vi "LoadPressureAndTangents.vi"(4 "error in (no error)":errorcluster, 5 "Red Graph":refnum<vi>, 6 "ResetFrontImage":bool, 7 "Blue Graph":refnum<vi>) -> (0 "error out":errorcluster, 3 "output cluster":cluster{dbl, dbl, dbl, dbl})   [LabVIEW 2013, in "main.lvlib"]
uses:
  main.lvlib
  Controls/Enum Process Data.ctl
  Controls/Combobox Filename.ctl
  Controls/Enum Variables.ctl
  <userlib>/_OpenG.lib/file/file.llb/File Exists - Scalar__ogtk.vi
  <vilib>/Utility/file.llb/Read From Spreadsheet File (DBL).vi
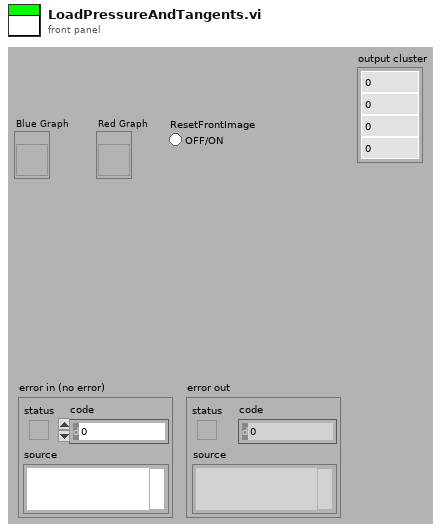
[diagram p1: front panel]
types:
  T1 = typedef "main.lvlib/Enum Variables.ctl" = enum16{"SetAcqFilter", "GetAcqFilter", "Set Filter", "Get Filter", "Set Height", "Get Height", "Set Recorded Height", "Get Recorded Height", "Set Blue Pressure", "Get Blue Pressure", "Set Red Pressure", "Get Red Pressure", "Init", "Reset Pressure", "Set Red Cursors", "Get Red Cursors", "Set Blue Cursors", "Get Blue Cursors", "Set Language", "Get Language", "Set Active Graphs", "Get ActiveGraphs", "Set Method", "Get Method", "Set Encryption", "Get Encryption", "Set ExcelVersion", "Get ExcelVersion", "Set DICOM Avail", "Get DICOM Avail", "Set DICOM Encode", "Get DICOM Encode", "Set JournalExport", "Get JournalExport", "Set Sequence", "Get Sequence", "Set DAQ Connected", "Get DAQ Connected", "Set Current Graph", "Get Current Graph", "Set General Settings", "Get Hyphenation", "Set Arm Calc Method", "Get Arm Calc Method", "Set Dicom Tags", "Get Dicom Tags", "Set BT Serial", "Get BT Serial", "Set BT Accepted Serials", "Get BT Accepted Serials", "Get BT License", "Set BT License"}
  T2 = typedef "main.lvlib/Combobox Filename.ctl" = string
  T3 = typedef "main.lvlib/Enum Process Data.ctl" = enum16{"Init", "Set Cursor Mode", "Set Data Path", "Get All"}
  T4 = cluster{dbl, dbl, "Armpressure":dbl, "Armpressure":dbl}
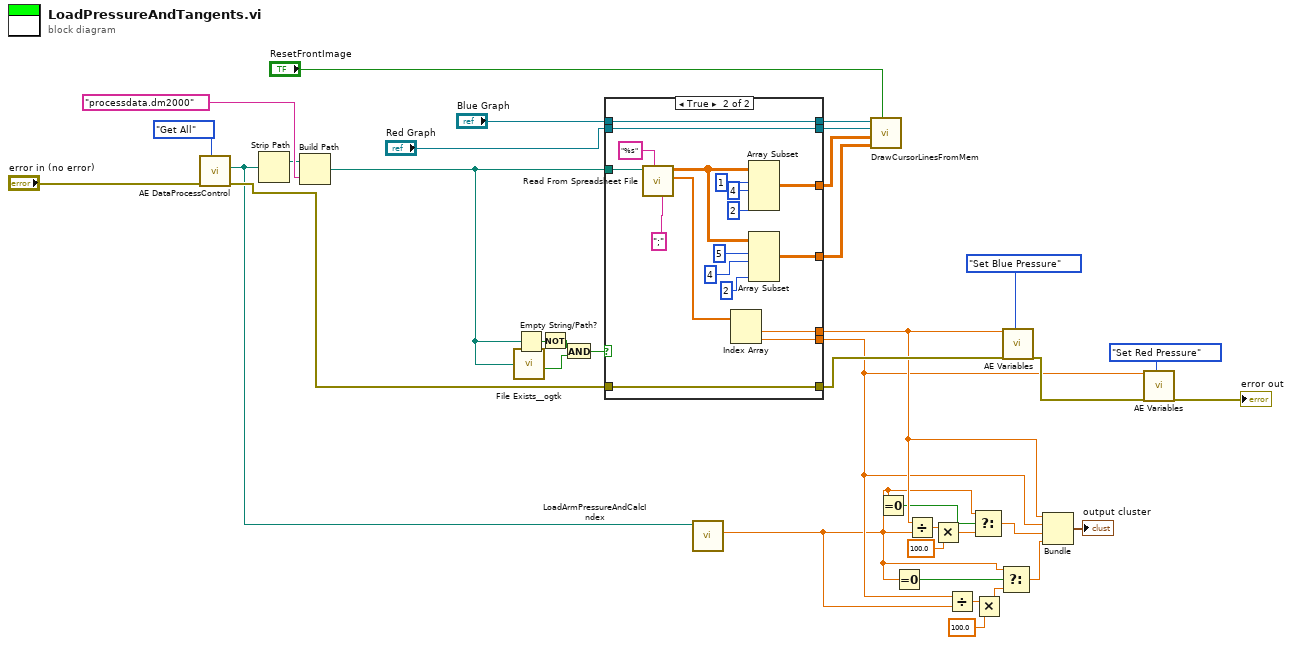
[diagram p0: block diagram]
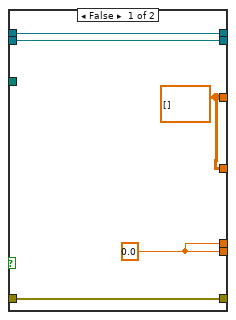
[diagram p2: hidden frame]
diagram:
  n1 = call "AE DataProcessControl.vi"("Action"=Enum_Process_Data."Get All", "error in (no error)"="error in (no error)") -> ("error out"=w25:errorcluster, "Data Path Out"=w21:path)  [unwired: 7 in, 1 out]
  n2 = Strip Path(path=w21) -> (stripped path=w28:path)  [unwired: 1 out]
  n3 = Build Path(base path=w28, name or relative path=T2 "processdata.dm2000" ("FileName")) -> (appended path=w1:path)
  n4 = call-poly <userlib>:"File Exists__ogtk.vi"("file path"=w1) -> ("exists"=w3:bool)  [unwired: 6 in, 1 out]
  n5 = Empty String/Path?(string/path=w1) -> (empty?=w5:bool)
  n6 = Not(x=w5) -> (.not. x?=w4:bool)
  n7 = And(x=w4, y=w3) -> (x .and. y?=w2:bool)
  n8 = case shown="True" w2 {
    tunnel: w1 -> [_ w57]
    tunnel: [w42 w56] -> w15
    tunnel: [w42 w55] -> w18
    tunnel: [w41 w51] -> w32
    tunnel: [w41 w49] -> w33
    tunnel: [w40 w45] -> w35
    tunnel: "Blue Graph" -> [w40 w45]
    tunnel: "Red Graph" -> [w39 w44]
    tunnel: [w39 w44] -> w36
    tunnel: w25 -> [w38 w43]
    tunnel: [w38 w43] -> w24
    frame False {
      w41 = dbl[][] []
      w42 = 0.0
    }
    frame True {
      n9 = call-poly <vilib>:"Read From Spreadsheet File.vi"("delimiter (\\t)"=";" ("delimiter (\\t)"), "format (%.3f)"="%s", "file path (dialog if empty)"=w57) -> ("first row"=w58:dbl[], "all rows"=w50:dbl[][])  [unwired: 4 in, 3 out]
      n10 = Index Array(array=w58) -> (element #1=w55:dbl, element #2=w56:dbl)  [unwired: 2 in]
      n11 = Array Subset(array=w50, index (row)=1 ("index"), length (row)=4 ("length"), length (col)=2 ("length")) -> (w51:dbl[][])  [unwired: 1 in]
      n12 = Array Subset(array=w50, index (row)=5 ("index"), length (row)=4 ("length"), length (col)=2 ("length")) -> (w49:dbl[][])  [unwired: 1 in]
    }
  }
  n13 = call "LoadArmPressureAndCalcIndex.vi"("Path"=w21) -> ("Armpressure"=w8:dbl)  [unwired: 8 in, 2 out]
  n14 = call "DrawCursorLinesFromMem.vi"("CursorMode"="ResetFrontImage", "RedPositionArray"=w33, "BluePositionArray"=w32, "Red"=w36, "Blue"=w35) -> ()  [unwired: 7 in]
  n15 = Equal To 0?(x=w8) -> (x = 0?=w13:bool)
  n16 = Equal To 0?(x=w8) -> (x = 0?=w10:bool)
  n17 = Divide(x=w18, y=w8) -> (x/y=w20:dbl)
  n18 = Multiply(x=w20, y=100.0) -> (x*y=w12:dbl)
  n19 = Divide(x=w15, y=w8) -> (x/y=w17:dbl)
  n20 = Select(t=w8, s=w13, f=w12) -> (s? t:f=w11:dbl)
  n21 = Multiply(x=w17, y=100.0) -> (x*y=w9:dbl)
  n22 = Select(t=w8, s=w10, f=w9) -> (s? t:f=w7:dbl)
  n23 = call "AE Variables.vi"("VariantIn"=w18, "error in (no error)"=w24, "Action"=Enum_Variables."Set Blue Pressure") -> ("error out"=w23:errorcluster)  [unwired: 9 in, 7 out]
  n24 = Bundle(w18, w15, "Armpressure"=w11, "Armpressure"=w7) -> (→"output cluster":T4)  [unwired: 1 in]
  n25 = call "AE Variables.vi"("VariantIn"=w15, "error in (no error)"=w23, "Action"=Enum_Variables."Set Red Pressure") -> ("error out"=→"error out":errorcluster)  [unwired: 9 in, 7 out]
